vi "UPortal Login.vi"(8 "error in":errorcluster, 9 "Password":string, 10 "User name":string="fedor@lanl.gov", 11 "Browser reference":refnum<k24>) -> (0 "error out":errorcluster, 3 "Browser reference out":refnum<k24>)   [LabVIEW 2020]
uses:
  System.Windows.Forms
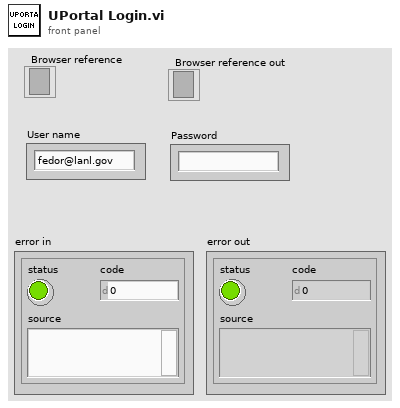
[diagram p1: front panel]
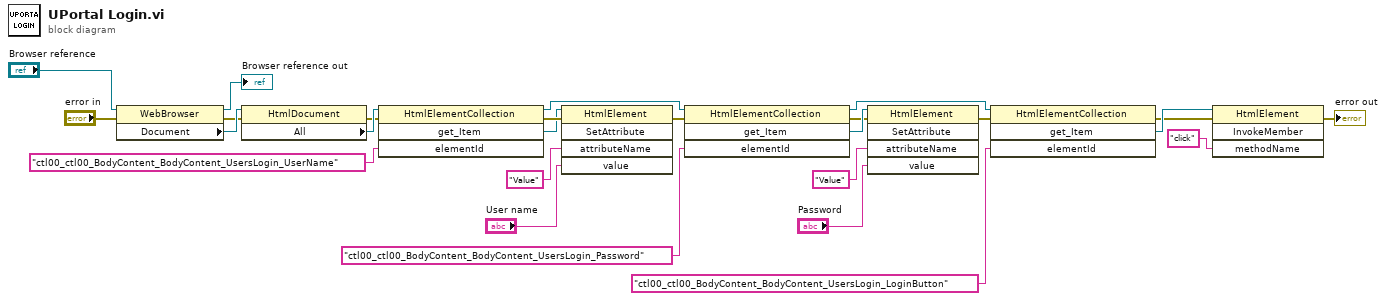
[diagram p0: block diagram]
diagram:
  n1 = property class="WebBrowser"(reference="Browser reference", error in="error in") -> (reference out=→"Browser reference out":refnum<k24>, error out=w24:errorcluster, "Document"=w25:refnum<k24>)
  n2 = property class="HtmlDocument"(reference=w25, error in=w24) -> (error out=w22:errorcluster, "All"=w23:refnum<k24>)  [unwired: 1 out]
  n3 = invoke class="HtmlElementCollection" method="get_Item"(reference=w23, error in=w22, "elementId"="ctl00_ctl00_BodyContent_BodyContent_UsersLogin_UserName") -> (reference out=w17:refnum<k24>, error out=w18:errorcluster, "get_Item"=w4:refnum<k24>)  [unwired: 1 in, 1 out]
  n4 = invoke class="HtmlElement" method="SetAttribute"(reference=w4, error in=w18, "attributeName"="Value", "value"="User name") -> (error out=w14:errorcluster)  [unwired: 1 in, 4 out]
  n5 = invoke class="HtmlElementCollection" method="get_Item"(reference=w17, error in=w14, "elementId"="ctl00_ctl00_BodyContent_BodyContent_UsersLogin_Password") -> (reference out=w9:refnum<k24>, error out=w11:errorcluster, "get_Item"=w13:refnum<k24>)  [unwired: 1 in, 1 out]
  n6 = invoke class="HtmlElement" method="SetAttribute"(reference=w13, error in=w11, "attributeName"="Value", "value"="Password") -> (error out=w6:errorcluster)  [unwired: 1 in, 4 out]
  n7 = invoke class="HtmlElementCollection" method="get_Item"(reference=w9, error in=w6, "elementId"="ctl00_ctl00_BodyContent_BodyContent_UsersLogin_LoginButton") -> (error out=w5:errorcluster, "get_Item"=w7:refnum<k24>)  [unwired: 1 in, 2 out]
  n8 = invoke class="HtmlElement" method="InvokeMember"(reference=w7, error in=w5, "methodName"="click" ("scriptName")) -> (error out=→"error out":errorcluster)  [unwired: 1 in, 3 out]
